vi "Get Refs APU Data.vi"(8 "error in (no error)":errorcluster, 10 "Label.Text":string, 11 "APU Setup":string[][](array[string])) -> (0 "error out":errorcluster, 3 "Thresold Array":dbl[](array[numeric]))   [LabVIEW 2018]
uses:
  Val Change Checker.vi
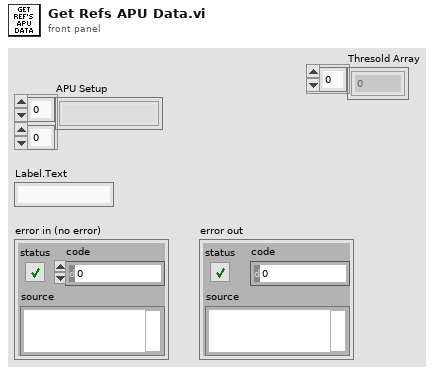
[diagram p1: front panel]
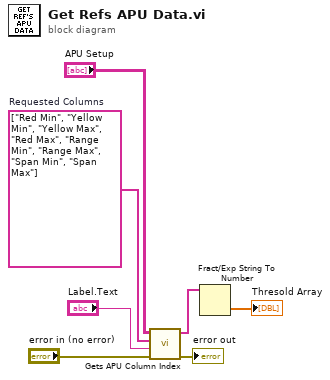
[diagram p0: block diagram]
diagram:
  w7 = string[] ["Red Min", "Yellow Min", "Yellow Max", "Red Max", "Range Min", "Range Max", "Span Min", "Span Max"]  # Requested Columns
  n1 = call "Gets APU Column Index.vi"("error in (no error)"="error in (no error)", "Tag"="Label.Text", "[Column Names]"=w7, "[[Array of Info]]"="APU Setup") -> ("error out"=→"error out":errorcluster, "[Values out]"=w1:string[])  [unwired: 3 in, 3 out]
  n2 = Fract/Exp String To Number(string=w1) -> (number=→"Thresold Array":dbl[])  [unwired: 3 in, 1 out]
